vi "defaultConfiguration.vi"(8 "error in (no error)":errorcluster, 11 "Xcite in":refnum<class "Xcite.lvclass">) -> (0 "error out":errorcluster, 3 "Xcite out":refnum<class "Xcite.lvclass">)   [LabVIEW 2019, in "Xcite.lvclass"]
doc: "Sets the XCite device to the default configuration, i.e. all channels off."
uses:
  Xcite.lvclass
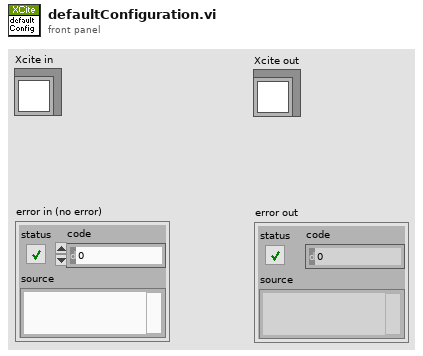
[diagram p1: front panel]
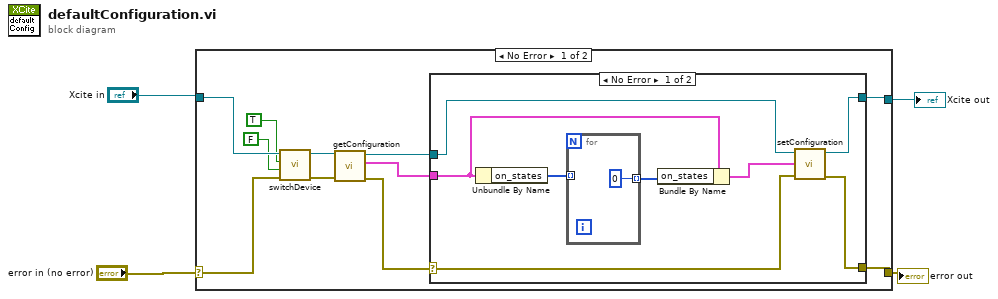
[diagram p0: block diagram]
diagram:
  n1 = case shown="No Error" "error in (no error)" {
    selector: "error in (no error)" -> [w7 w28]
    tunnel: [w13 w28] -> w3
    tunnel: "Xcite in" -> [w10 w27]
    tunnel: [w11 w27] -> w1
    frame No Error {
      n2 = call "switchDevice.vi"("error in (no error)"=w7, "on"=FALSE, "use_common_on_off"=TRUE, "Xcite in"=w10) -> ("error out"=w8:errorcluster, "Xcite out"=w9:refnum<class "Xcite.lvclass">)  [unwired: 6 in]
      n3 = call "getConfiguration.vi"("error in (no error)"=w8, "Xcite in"=w9) -> ("error out"=w15:errorcluster, "configuration"=w12:cluster{"intensities":u32[], "on_states":u8[]}, "Xcite out"=w14:refnum<class "Xcite.lvclass">)  [unwired: 7 in]
      n4 = case shown="No Error" w15 {
        selector: w15 -> [w23 w26]
        tunnel: w14 -> [w20 w25]
        tunnel: [w22 w26] -> w13
        tunnel: w12 -> [w18 _]
        tunnel: [w19 w25] -> w11
        frame No Error {
          n5 = Unbundle By Name(w18) -> ("on_states"=w21:u8[])
          n6 = for {
            tunnel: w21 -> [_] mode=indexing
            tunnel: [u8 0 ("Numeric")] -> w17 mode=indexing
          }
          n7 = Bundle By Name(cluster=w18, "on_states"=w17) -> (w16:cluster{"intensities":u32[], "on_states":u8[]})
          n8 = call "setConfiguration.vi"("error in (no error)"=w23, "configuration"=w16, "Xcite in"=w20) -> ("error out"=w22:errorcluster, "Xcite out"=w19:refnum<class "Xcite.lvclass">)  [unwired: 7 in]
        }
        frame Error {
        }
      }
    }
    frame Error {
    }
  }
  "Xcite out" <- w1
  "error out" <- w3
